vi "Script Add Custom Error -- Project.vi"(4 "Selection Owning Folder":path, 5 "Error Code":i32, 6 "Error Description":string, 7 "Error Name":string="TESTING.vi", 8 "error in":errorcluster, 9 "Error Arguments Window Ref":refnum<vi>, 10 "Project Reference":refnum<vi>) -> (0 "error out":errorcluster, 3 "Error VI Path":path)   [LabVIEW 2020, in "ConstantErrorsMaker.lvlib"]
uses:
  ConstantErrorsMaker.lvlib
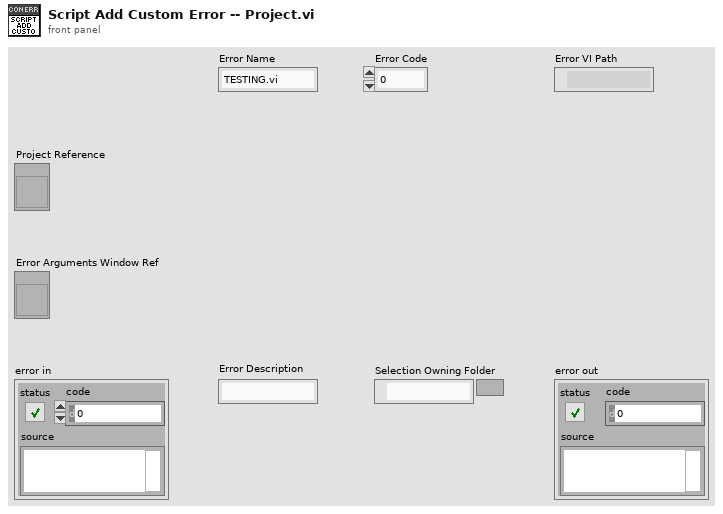
[diagram p1: front panel]
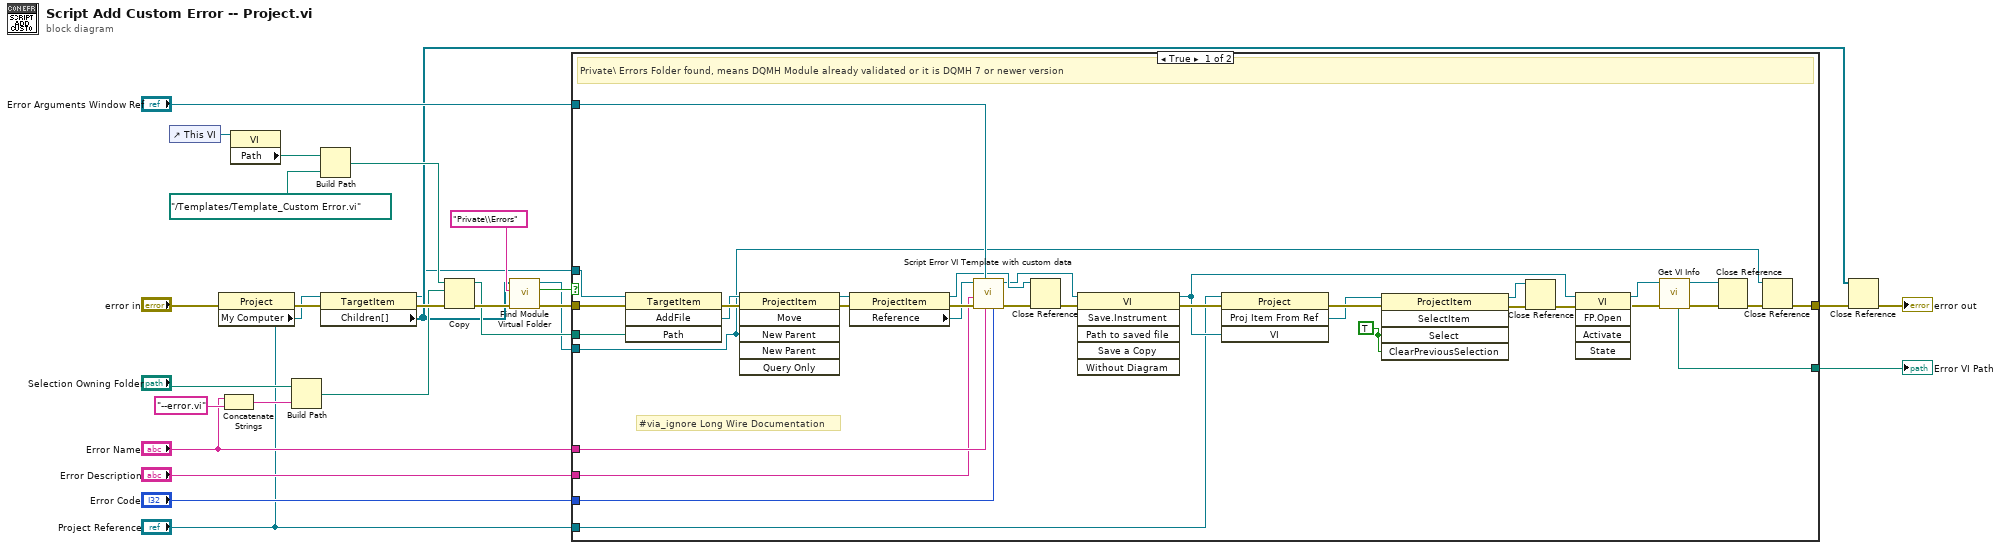
[diagram p0: block diagram]
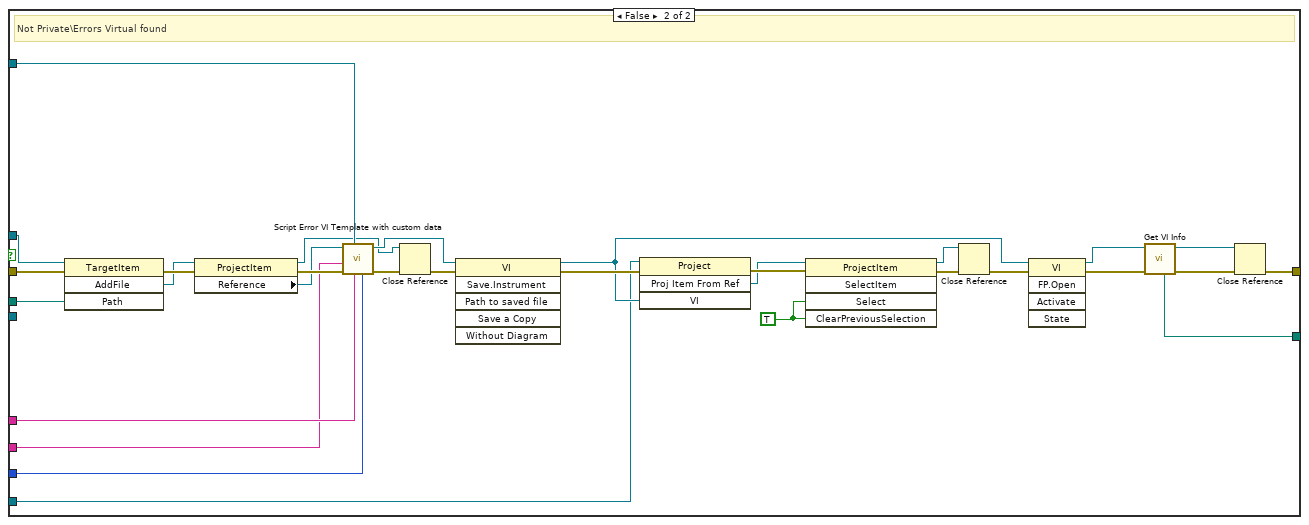
[diagram p2: hidden frame]
diagram:
  n1 = control-ref of="This VI"() -> (w19:refnum<vi>)
  n2 = property class="Project"(reference="Project Reference", error in="error in") -> (error out=w23:errorcluster, "My Computer"=w4:refnum<vi>)  [unwired: 1 out]
  n3 = Concatenate Strings("Error Name", "--error.vi" ("input 1")) -> (w21:string)
  n4 = property class="VI"(reference=w19) -> ("Path"=w18:path)  [unwired: 1 in, 2 out]
  n5 = Build Path(base path="Selection Owning Folder", name or relative path=w21) -> (appended path=w20:path)
  n6 = Build Path(base path=w18, name or relative path=path "../Templates/Template_Custom Error.vi") -> (appended path=w16:path)
  n7 = property class="TargetItem"(reference=w4, error in=w23) -> (reference out=w3:refnum<vi>, error out=w24:errorcluster, "Children[]"=w5:refnum<vi>[])
  n8 = Copy(8:w24, 10:w20, 11:w16) -> (0:w25:errorcluster, 3:w14:path)  [unwired: 2 in, 1 out]
  n9 = call "Find Module Virtual Folder.vi"("error in"=w25, "Virtual Folder"="Private\\Errors", "Children"=w5) -> ("error out"=w26:errorcluster, "Found?"=w9:bool, "ProjectItem out"=w8:refnum<vi>)  [unwired: 6 in]
  n10 = case shown="True" w9 {
    tunnel: [w60 w89] -> w28
    tunnel: w3 -> [w49 w80]
    tunnel: w14 -> [w50 w81]
    tunnel: "Error Name" -> [w43 w76]
    tunnel: "Error Code" -> [w46 w78]
    tunnel: "Error Arguments Window Ref" -> [w45 w77]
    tunnel: "Error Description" -> [w41 w74]
    tunnel: w8 -> [w40 _]
    tunnel: w26 -> [w57 w83]
    tunnel: "Project Reference" -> [w36 w68]
    tunnel: [w29 w63] -> w1
    frame True {
      w37 = TRUE ("Select")
      # "#via_ignore Long Wire Documentation"
      # "Private\\ Errors Folder found, means DQMH Module already validated or it is DQMH 7 or newer version"
      n11 = invoke class="TargetItem" method="AddFile"(reference=w49, error in=w57, "Path"=w50) -> (error out=w61:errorcluster, "AddFile"=w48:refnum<vi>)  [unwired: 1 in, 2 out]
      n12 = invoke class="ProjectItem" method="Move"(reference=w48, error in=w61, "New Parent"=w40) -> (reference out=w47:refnum<vi>, error out=w62:errorcluster)  [unwired: 3 in, 4 out]
      n13 = property class="ProjectItem"(reference=w47, error in=w62) -> (reference out=w44:refnum<vi>, error out=w51:errorcluster, "Reference"=w34:refnum<vi>)
      n14 = call "Script Error VI Template with custom data.vi"("Error Code"=w46, "Error Name"=w43, "Error Arguments Window Ref"=w45, "error in"=w51, "Error Description"=w41, "VI Ref Error in"=w34) -> ("error out"=w53:errorcluster, "Custom Error VI Ref"=w42:refnum<vi>)  [unwired: 4 in]
      n15 = Close Reference(reference=w44, error in (no error)=w53) -> (error out=w59:errorcluster)
      n16 = invoke class="VI" method="Save.Instrument"(reference=w42, error in=w59) -> (reference out=w39:refnum<vi>, error out=w56:errorcluster)  [unwired: 4 in, 4 out]
      n17 = invoke class="Project" method="Proj Item From Ref"(reference=w36, error in=w56, "VI"=w39) -> (error out=w55:errorcluster, "ProjItemFromRef"=w38:refnum<vi>)  [unwired: 1 in, 2 out]
      n18 = invoke class="ProjectItem" method="SelectItem"(reference=w38, error in=w55, "Select"=w37, "ClearPreviousSelection"=w37) -> (reference out=w35:refnum<vi>, error out=w54:errorcluster)  [unwired: 1 in, 3 out]
      n19 = Close Reference(reference=w35, error in (no error)=w54) -> (error out=w52:errorcluster)
      n20 = invoke class="VI" method="FP.Open"(reference=w39, error in=w52) -> (reference out=w31:refnum<vi>, error out=w33:errorcluster)  [unwired: 3 in, 3 out]
      n21 = call "Get VI Info.vi"("error in"=w33, "VI in"=w31) -> ("error out"=w32:errorcluster, "VI out"=w30:refnum<vi>, "VI Path"=w29:path)  [unwired: 4 in, 3 out]
      n22 = Close Reference(reference=w30, error in (no error)=w32) -> (error out=w58:errorcluster)
      n23 = Close Reference(reference=w40, error in (no error)=w58) -> (error out=w60:errorcluster)
    }
    frame False {
      w72 = TRUE ("Select")
      # "Not Private\\Errors Virtual found"
      n24 = invoke class="TargetItem" method="AddFile"(reference=w80, error in=w83, "Path"=w81) -> (error out=w92:errorcluster, "AddFile"=w79:refnum<vi>)  [unwired: 1 in, 2 out]
      n25 = property class="ProjectItem"(reference=w79, error in=w92) -> (reference out=w67:refnum<vi>, error out=w82:errorcluster, "Reference"=w69:refnum<vi>)
      n26 = call "Script Error VI Template with custom data.vi"("Error Code"=w78, "Error Name"=w76, "Error Arguments Window Ref"=w77, "error in"=w82, "Error Description"=w74, "VI Ref Error in"=w69) -> ("error out"=w85:errorcluster, "Custom Error VI Ref"=w75:refnum<vi>)  [unwired: 4 in]
      n27 = Close Reference(reference=w67, error in (no error)=w85) -> (error out=w91:errorcluster)
      n28 = invoke class="VI" method="Save.Instrument"(reference=w75, error in=w91) -> (reference out=w71:refnum<vi>, error out=w87:errorcluster)  [unwired: 4 in, 4 out]
      n29 = invoke class="Project" method="Proj Item From Ref"(reference=w68, error in=w87, "VI"=w71) -> (error out=w88:errorcluster, "ProjItemFromRef"=w73:refnum<vi>)  [unwired: 1 in, 2 out]
      n30 = invoke class="ProjectItem" method="SelectItem"(reference=w73, error in=w88, "Select"=w72, "ClearPreviousSelection"=w72) -> (reference out=w70:refnum<vi>, error out=w86:errorcluster)  [unwired: 1 in, 3 out]
      n31 = Close Reference(reference=w70, error in (no error)=w86) -> (error out=w84:errorcluster)
      n32 = invoke class="VI" method="FP.Open"(reference=w71, error in=w84) -> (reference out=w65:refnum<vi>, error out=w90:errorcluster)  [unwired: 3 in, 3 out]
      n33 = call "Get VI Info.vi"("error in"=w90, "VI in"=w65) -> ("error out"=w66:errorcluster, "VI out"=w64:refnum<vi>, "VI Path"=w63:path)  [unwired: 4 in, 3 out]
      n34 = Close Reference(reference=w64, error in (no error)=w66) -> (error out=w89:errorcluster)
    }
  }
  "Error VI Path" <- w1
  n35 = Close Reference(reference=w5, error in (no error)=w28) -> (error out=→"error out":errorcluster)
